vi "Save Motion Profile.vi"(8 "error in (no error)":errorcluster, 10 "File Path (.csv)":path, 11 "Motion Profile Generator in":refnum<class "Motion Profile Generator.lvclass">) -> (0 "error out":errorcluster, 2 "New File Path (.csv)":path, 3 "Motion Profile Generator out":refnum<class "Motion Profile Generator.lvclass">)   [LabVIEW 2019, in "Motion Profile Generator.lvclass"]
uses:
  Motion Profile Generator.lvclass
  Motion Profile Generator.lvclass/Motion Profile Generator.ctl
  <vilib>/Utility/file.llb/Write Delimited Spreadsheet (DBL).vi
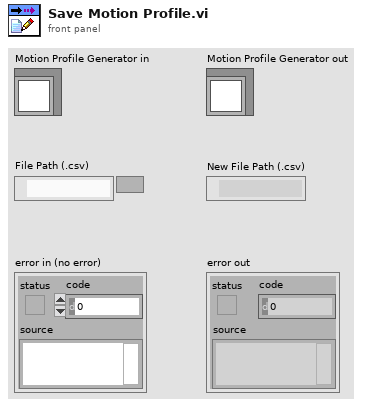
[diagram p1: front panel]
types:
  T1 = typedef "Motion Profile Generator.lvclass/Motion Profile Point.ctl" = cluster{"Position (in)":dbl, "Velocity (in/s)":dbl, "Duration (ms)":dbl}
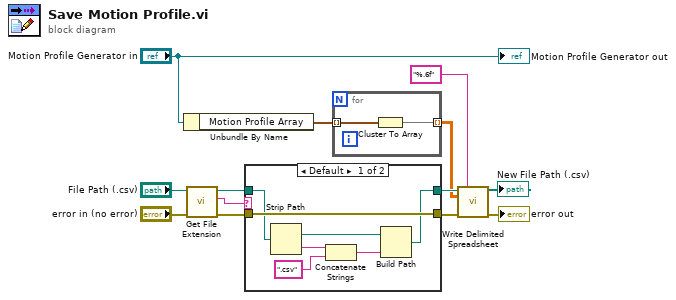
[diagram p0: block diagram]
diagram:
  n1 = Unbundle By Name("Motion Profile Generator in") -> ("Motion Profile Array"=w2:T1[])
  n2 = call <vilib>:"Get File Extension.vi"("error in (no error)"="error in (no error)", "file"="File Path (.csv)") -> ("error out"=w7:errorcluster, "lowercase file extension"=w11:string, "dup file"=w10:path)  [unwired: 5 in, 2 out]
  n3 = case shown="Default" w11 {
    tunnel: w10 -> [w14 w21]
    tunnel: [w20 w22] -> w8
    tunnel: w7 -> [w20 w22]
    tunnel: [w15 w21] -> w5
    frame Default {
      n4 = Strip Path(path=w14) -> (stripped path=w16:path, name=w19:string)
      n5 = Concatenate Strings(w19, ".csv" ("string")) -> (w17:string)
      n6 = Build Path(base path=w16, name or relative path=w17) -> (appended path=w15:path)
    }
    frame "csv" {
    }
  }
  n7 = for {
    tunnel: w2 -> [w24] mode=indexing
    tunnel: [w23] -> w1 mode=indexing
    n8 = Cluster To Array(cluster=w24) -> (array=w23:dbl[])
  }
  n9 = call-poly <vilib>:"Write Delimited Spreadsheet.vi"("file path (dialog if empty)"=w5, "format (%.3f)"="%.6f", "2D data"=w1, "error in (no error)"=w8) -> ("new file path (Not A Path if cancelled)"=→"New File Path (.csv)":path, "error out"=→"error out":errorcluster)  [unwired: 10 in]
  "Motion Profile Generator out" <- "Motion Profile Generator in"
